vi "Template_MouseDown.vi"(7 "Add to Undo?":bool=TRUE, 8 "error in":errorcluster, 10 "CtlRef":refnum<vi>, 11 "Data in":T1={"Class"={"Ants"=refnum, "Layer"=refnum, "Templates"=refnum, "Icon"=refnum, "Glyph"=refnum, "Settings"=refnum, "Tools"=refnum}, "Ref"={"Add Layer"=refnum, "Remove Layer"=refnum, "Line Text"=[], "Body Text Spec"=refnum, "DNL_Font"=refnum, "glyph path str"=refnum, "templates path str"=refnum, "Arrow Up"=refnum, "Arrow Down"=refnum, "IE VI Ref"=refnum, "Glyphs tree"=refnum, "Templates tree"=refnum, "Layer Icon Text"=refnum, "Layer Template"=refnum, "Clipboard"=refnum, "BW icon in"=refnum, "Color icon in"=refnum, "Layer Clust"=refnum, "Body Text"=refnum, "DNL_Framework Templates"=refnum, "Search Templates"=refnum, "TextMarker"=refnum, "Tab Control"=refnum, "Search Glyphs"=refnum, "Line Color"=refnum, "DNL_Glyphs []"=refnum, "Fill Color"=refnum, "Tools"=refnum, "Glyphs tree"=refnum, "Icon"=refnum, "Preview"=refnum, "Ants"=refnum, "Terminals"=refnum, "menu reference"=refnum, "LayerNames"=[], "GlyphLoadAnimation"=refnum, "TemplateLoadAnimation"=refnum, "refreshGlyphs"=refnum, "refreshTemplates"=refnum}, "Support"={"AntsRect"={"left"=0, "top"=0, "right"=0, "bottom"=0}, "Mouse Move Coords"={"Horizontal"=0, "Vertical"=0}, "Mouse Down Coords"={"Horizontal"=0, "Vertical"=0}, "Temp Coord"={"Horizontal"=0, "Vertical"=0}, "Action"=enum."Default", "Edge Color"=4914962, "Fill Color"=16860, "Mouse Down?"=FALSE, "Draft Mode?"=FALSE, "Temp Icon"=bytes[3102], "CTRL Pressed"=FALSE, "Move Selection?"=FALSE, "AntsRect Orig"={"left"=0, "top"=0, "right"=0, "bottom"=0}, "Text"="", "TM Set?"=FALSE, "Mouse inside icon?"=FALSE, "Tool (old value)"=0, "Pencil Move Color"=0, "Swap Colors?"=FALSE, "Shift pressed?"=FALSE}}) -> (0 "error out":errorcluster, 3 "Data out":T1={"Class"={"Ants"=refnum, "Layer"=refnum, "Templates"=refnum, "Icon"=refnum, "Glyph"=refnum, "Settings"=refnum, "Tools"=refnum}, "Ref"={"Add Layer"=refnum, "Remove Layer"=refnum, "Line Text"=[], "Body Text Spec"=refnum, "DNL_Font"=refnum, "glyph path str"=refnum, "templates path str"=refnum, "Arrow Up"=refnum, "Arrow Down"=refnum, "IE VI Ref"=refnum, "Glyphs tree"=refnum, "Templates tree"=refnum, "Layer Icon Text"=refnum, "Layer Template"=refnum, "Clipboard"=refnum, "BW icon in"=refnum, "Color icon in"=refnum, "Layer Clust"=refnum, "Body Text"=refnum, "DNL_Framework Templates"=refnum, "Search Templates"=refnum, "TextMarker"=refnum, "Tab Control"=refnum, "Search Glyphs"=refnum, "Line Color"=refnum, "DNL_Glyphs []"=refnum, "Fill Color"=refnum, "Tools"=refnum, "Glyphs tree"=refnum, "Icon"=refnum, "Preview"=refnum, "Ants"=refnum, "Terminals"=refnum, "menu reference"=refnum, "LayerNames"=[], "GlyphLoadAnimation"=refnum, "TemplateLoadAnimation"=refnum, "refreshGlyphs"=refnum, "refreshTemplates"=refnum}, "Support"={"AntsRect"={"left"=0, "top"=0, "right"=0, "bottom"=0}, "Mouse Move Coords"={"Horizontal"=0, "Vertical"=0}, "Mouse Down Coords"={"Horizontal"=0, "Vertical"=0}, "Temp Coord"={"Horizontal"=0, "Vertical"=0}, "Action"=enum."Default", "Edge Color"=4914962, "Fill Color"=16860, "Mouse Down?"=FALSE, "Draft Mode?"=FALSE, "Temp Icon"=bytes[3102], "CTRL Pressed"=FALSE, "Move Selection?"=FALSE, "AntsRect Orig"={"left"=0, "top"=0, "right"=0, "bottom"=0}, "Text"="", "TM Set?"=FALSE, "Mouse inside icon?"=FALSE, "Tool (old value)"=0, "Pencil Move Color"=0, "Swap Colors?"=FALSE, "Shift pressed?"=FALSE}})   [LabVIEW 2021]
uses:
  Controls/IE Data.ctl
  Class/Ants/Ants.lvclass
  Class/FakedArray/FakedArray.lvclass
  vi.lib/LabVIEW Icon API/lv_icon/Classes/Icon/Icon.lvclass
  Class/Icon Library/Glyph.lvclass
  Class/Settings/Settings.lvclass
  Class/Tools/Tools Paint.lvclass
  Controls/IE Classes.ctl
  Controls/References Cluster.ctl
  Controls/SupportClass.ctl
  <vilib>/Utility/miscctls.llb/LVPoint32TypeDef.ctl
  Controls/SupportClass_Action.ctl
  vi.lib/LabVIEW Icon API/lv_icon/Controls/IEColor.ctl
  vi.lib/LabVIEW Icon API/lv_icon/Controls/LayerType.ctl
  vi.lib/LabVIEW Icon API/lv_icon/Classes/Icon Framework/Icon Framework.lvclass
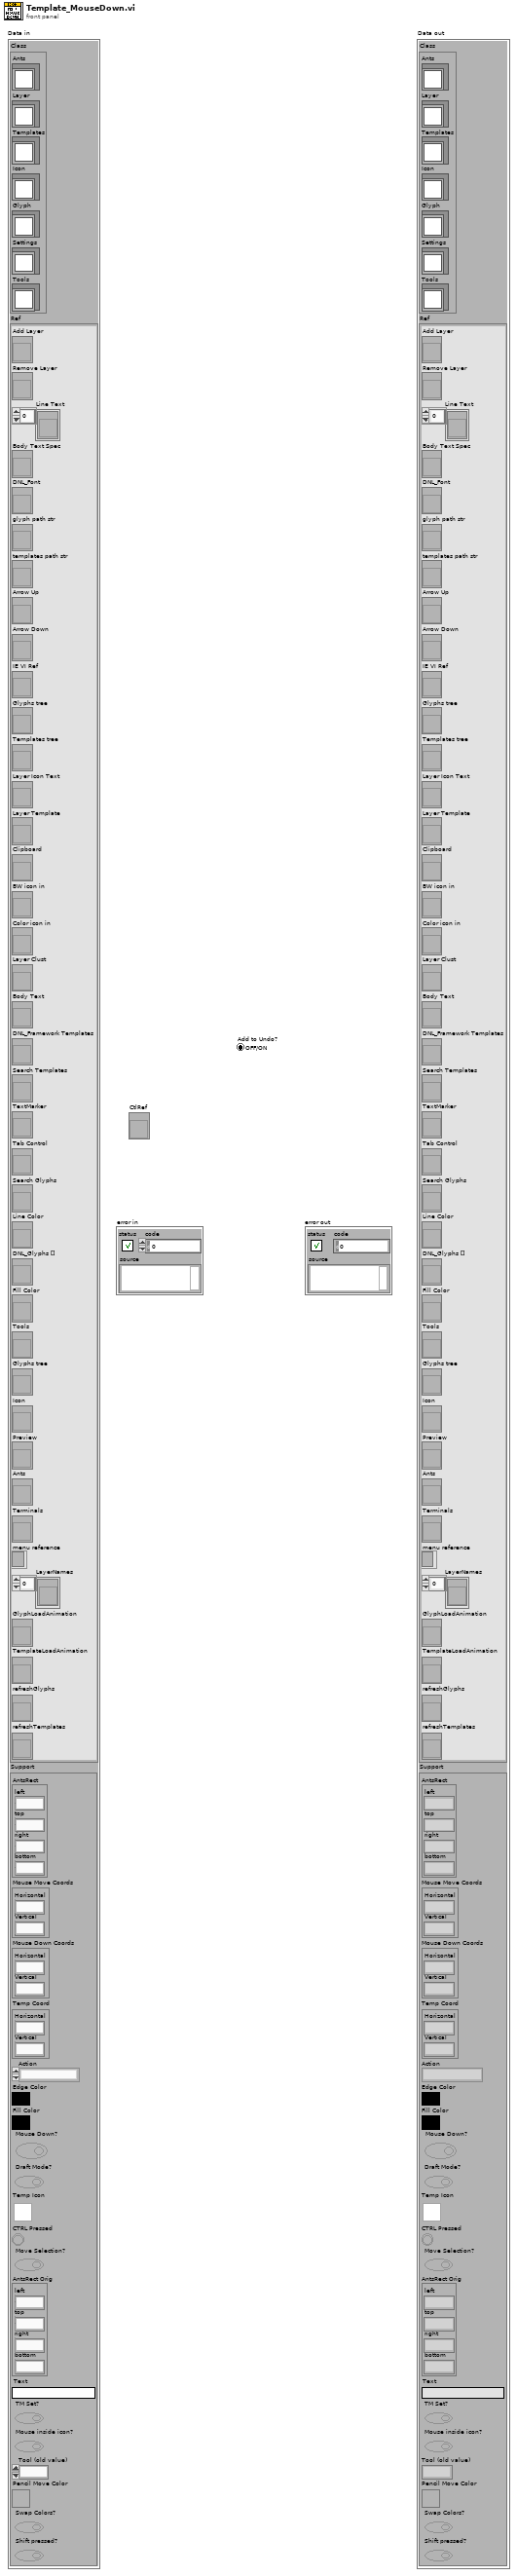
[diagram p1: front panel]
types:
  T1 = typedef "IE Data.ctl" = cluster{"Class":T2, "Ref":T3, "Support":T4}
  T2 = typedef "IE Classes.ctl" = cluster{"Ants":refnum<class "Ants.lvclass">, "Layer":refnum<class "FakedArray.lvclass">, "Templates":refnum<class "FakedArray.lvclass">, "Icon":refnum<class "Icon.lvclass">, "Glyph":refnum<class "Glyph.lvclass">, "Settings":refnum<class "Settings.lvclass">, "Tools":refnum<class "Tools Paint.lvclass">}
  T3 = typedef "References Cluster.ctl" = cluster{"Add Layer":refnum<vi>, "Remove Layer":refnum<vi>, "Line Text":refnum<vi>[], "Body Text Spec":refnum<vi>, "DNL_Font":refnum<vi>, "glyph path str":refnum<vi>, "templates path str":refnum<vi>, "Arrow Up":refnum<vi>, "Arrow Down":refnum<vi>, "IE VI Ref":refnum<vi>, "Glyphs tree":refnum<vi>, "Templates tree":refnum<vi>, "Layer Icon Text":refnum<vi>, "Layer Template":refnum<vi>, "Clipboard":refnum<vi>, "BW icon in":refnum<vi>, "Color icon in":refnum<vi>, "Layer Clust":refnum<vi>, "Body Text":refnum<vi>, "DNL_Framework Templates":refnum<vi>, "Search Templates":refnum<vi>, "TextMarker":refnum<vi>, "Tab Control":refnum<vi>, "Search Glyphs":refnum<vi>, "Line Color":refnum<vi>, "DNL_Glyphs []":refnum<vi>, "Fill Color":refnum<vi>, "Tools":refnum<vi>, "Glyphs tree":refnum<vi>, "Icon":refnum<vi>, "Preview":refnum<vi>, "Ants":refnum<vi>, "Terminals":refnum<vi>, "menu reference":refnum<k9>, "LayerNames":refnum<vi>[], "GlyphLoadAnimation":refnum<vi>, "TemplateLoadAnimation":refnum<vi>, "refreshGlyphs":refnum<vi>, "refreshTemplates":refnum<vi>}
  T4 = typedef "SupportClass.ctl" = cluster{"AntsRect":cluster{"left":i16, "top":i16, "right":i16, "bottom":i16}, "Mouse Move Coords":T5, "Mouse Down Coords":T5, "Temp Coord":T5, "Action":T6, "Edge Color":T7, "Fill Color":T7, "Mouse Down?":bool, "Draft Mode?":bool, "Temp Icon":picture, "CTRL Pressed":bool, "Move Selection?":bool, "AntsRect Orig":cluster{"left":i16, "top":i16, "right":i16, "bottom":i16}, "Text":string, "TM Set?":bool, "Mouse inside icon?":bool, "Tool (old value)":u32, "Pencil Move Color":u32, "Swap Colors?":bool, "Shift pressed?":bool}
  T5 = typedef "LVPoint32TypeDef.ctl" = cluster{"Horizontal":i32, "Vertical":i32}
  T6 = typedef "SupportClass_Action.ctl" = enum16{"Default", "Move Selection", "Glyph Library", "Tool"}
  T7 = typedef "IEColor.ctl" = u32
  T8 = typedef "LayerType.ctl" = enum16{"Graphic", "Text", "Tool", "Graphic Drop"}
  T9 = typedef "Graphic.ctl" = cluster{"Rectangle":cluster{"left":i16, "top":i16, "right":i16, "bottom":i16}, "Path":path, "Image":picture, "Filter":string, "FileName":string}
  T10 = typedef "Layer.ctl" = cluster{"LayerIcon":picture, "LayerName":string, "Opacity":u8, "Visibility?":bool}
  T11 = typedef "Font.ctl" = string
  T12 = typedef "Alignment.ctl" = u16
  T13 = typedef "Font Size.ctl" = u8
  T14 = cluster{"Line 1 text":string, "Line 2 text":string, "Line 3 text":string, "Line 4 text":string, "Line 1 color":u32, "Line 2 color":u32, "Line 3 color":u32, "Line 4 color":u32, "Body Text Spec":cluster{"DNL_Font":T11, "Alignment":T12, "Size":T13}, "Center text vertically":bool, "Capitalize Text":bool}
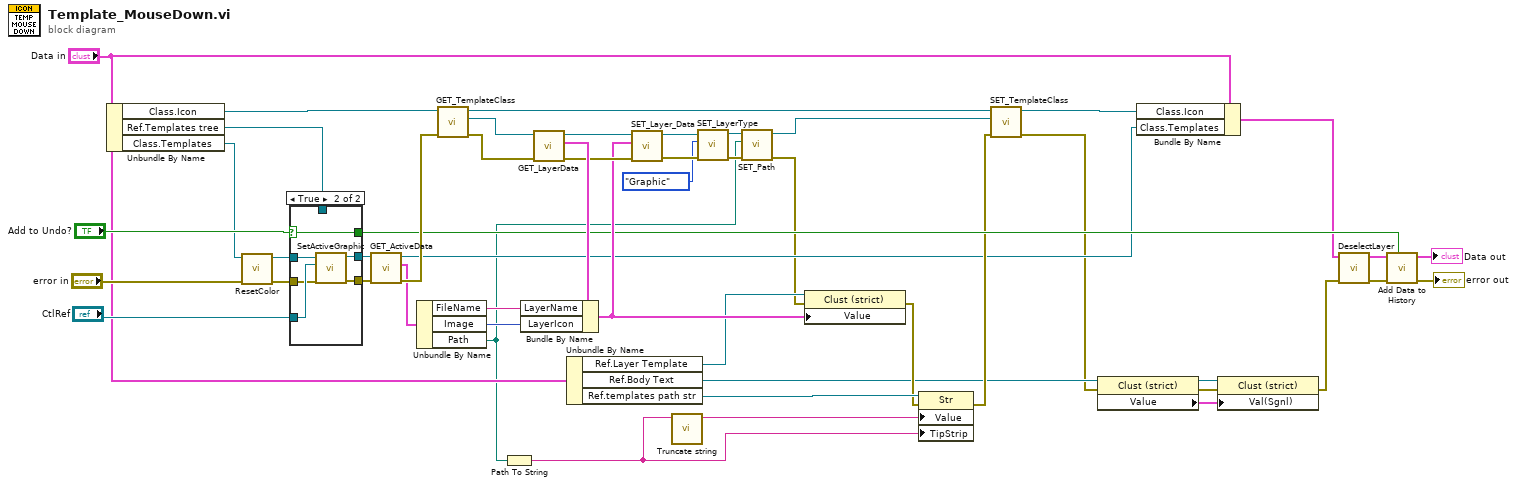
[diagram p0: block diagram]
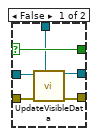
[diagram p2: hidden frame]
diagram:
  n1 = Unbundle By Name("Data in") -> ("Class.Icon"=w17:refnum<class "Icon.lvclass">, "Ref.Templates tree"=w6:refnum<vi>, "Class.Templates"=w15:refnum<class "FakedArray.lvclass">)
  n2 = call "ResetColor.vi"("error in (no error)"="error in", "FakedArray in"=w15) -> ("error out"=w35:errorcluster, "FakedArray out"=w36:refnum<class "FakedArray.lvclass">)  [unwired: 8 out]
  n3 = case shown="True" "Add to Undo?" {
    selector: "Add to Undo?" -> [w54 w57]
    tunnel: "CtlRef" -> [_ w62]
    tunnel: [w53 w61] -> w49
    tunnel: [w55 w60] -> w48
    tunnel: w36 -> [w52 w59]
    tunnel: w35 -> [w56 w58]
    tunnel: [w54 w57] -> w28
    tunnel: w6 -> [w51 _]
    frame False {
      n4 = call-dynamic "UpdateVisibleData.vi"("Templates tree"=w51, "error in (no error)"=w56, "FakedArray in"=w52) -> ("error out"=w55:errorcluster, "FakedArray out"=w53:refnum<class "FakedArray.lvclass">)  [unwired: 2 in, 5 out]
    }
    frame True {
      n5 = call-dynamic "SetActiveGraphic.vi"("error in (no error)"=w58, "Ctl Refnum"=w62, "FakedArray in"=w59) -> ("error out"=w60:errorcluster, "FakedArray out"=w61:refnum<class "FakedArray.lvclass">)  [unwired: 3 in, 4 out]
    }
  }
  n6 = call-dynamic "GET_ActiveData.vi"("error in (no error)"=w48, "FakedArray in"=w49) -> ("error out"=w39:errorcluster, "Path & Icon"=w32:T9, "FakedArray out"=w14:refnum<class "FakedArray.lvclass">)  [unwired: 7 out]
  n7 = Unbundle By Name(w32) -> ("FileName"=w23:string, "Image"=w47:picture, "Path"=w1:path)
  n8 = call-dynamic "GET_TemplateClass.vi"("error in (no error)"=w39, "Icon.lvclass in"=w17) -> ("error out"=w34:errorcluster, "Icon Framework.lvclass"=w37:refnum<class "Icon Framework.lvclass">, "Icon.lvclass out"=w40:refnum<class "Icon.lvclass">)  [unwired: 7 out]
  n9 = Path To String(path=w1) -> (string=w22:string)
  n10 = call-dynamic "GET_LayerData.vi"("error in (no error)"=w34, "Layer.lvclass in"=w37) -> ("error out"=w41:errorcluster, "Data"=w42:T10, "Layer.lvclass out"=w43:refnum<class "Icon Framework.lvclass">)  [unwired: 7 out]
  n11 = Bundle By Name(cluster=w42, "LayerName"=w23, "LayerIcon"=w47) -> (w38:T10)
  n12 = Unbundle By Name("Data in") -> ("Ref.Layer Template"=w33:refnum<vi>, "Ref.Body Text"=w21:refnum<vi>, "Ref.templates path str"=w27:refnum<vi>)
  n13 = call-dynamic "SET_Layer_Data.vi"("error in (no error)"=w41, "Data"=w38, "Layer.lvclass in"=w43) -> ("error out"=w46:errorcluster, "Layer.lvclass out"=w44:refnum<class "Icon Framework.lvclass">)  [unwired: 1 in, 6 out]
  n14 = call "Truncate string.vi"("String Path in"=w22) -> ("String path out"=w24:string)  [unwired: 1 in, 9 out]
  n15 = call-dynamic "SET_LayerType.vi"("error in (no error)"=w46, "Type"=LayerType."Graphic", "Layer.lvclass in"=w44) -> ("error out"=w3:errorcluster, "Layer.lvclass out"=w5:refnum<class "Icon Framework.lvclass">)  [unwired: 7 out]
  n16 = call "SET_Path.vi"("error in (no error)"=w3, "Path"=w1, "Icon Framework.lvclass in"=w5) -> ("error out"=w2:errorcluster, "Icon Framework.lvclass out"=w4:refnum<class "Icon Framework.lvclass">)  [unwired: 7 in]
  n17 = property class="Clust (strict)"(reference=w33, error in=w2, "Value"=w38) -> (error out=w26:errorcluster)  [unwired: 1 out]
  n18 = property class="Str"(reference=w27, error in=w26, "Value"=w24, "TipStrip"=w22) -> (error out=w25:errorcluster)  [unwired: 1 out]
  n19 = call-dynamic "SET_TemplateClass.vi"("error in (no error)"=w25, "Icon Framework.lvclass"=w4, "Icon.lvclass in"=w40) -> ("error out"=w13:errorcluster, "Icon.lvclass out"=w16:refnum<class "Icon.lvclass">)  [unwired: 7 out]
  n20 = property class="Clust (strict)"(reference=w21, error in=w13) -> (reference out=w20:refnum<vi>, error out=w19:errorcluster, "Value"=w18:T14)
  n21 = Bundle By Name(cluster="Data in", "Class.Icon"=w16, "Class.Templates"=w14) -> (w11:T1)
  n22 = property class="Clust (strict)"(reference=w20, error in=w19, "Val(Sgnl)"=w18) -> (error out=w12:errorcluster)  [unwired: 1 out]
  n23 = call "DeselectLayer.vi"("error in (no error)"=w12, "Data in"=w11) -> ("error out"=w31:errorcluster, "Data out"=w10:T1)  [unwired: 8 out]
  n24 = call "Add Data to History.vi"("Add to Undo?"=w28, "error in"=w31, "Data in"=w10) -> ("error out"=→"error out":errorcluster, "Data out"=→"Data out":T1)  [unwired: 7 out]
